vi "CgStop.vi"(3 "error in (no error)":errorcluster, 5 "VISA resource name":refnum<visa-resource-name>) -> (0 "error out":errorcluster, 2 "VISA resource name out":refnum<visa-resource-name>)   [LabVIEW 2009]
doc: "Stops streaming mode of the cyberglove. Also clears any brewing problems with input (at least mostly). Turns light off as well to signal that it is not recording."
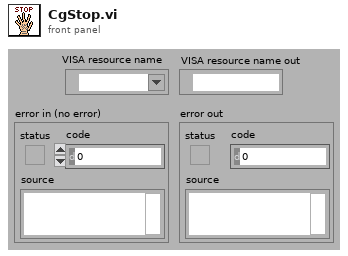
[diagram p1: front panel]
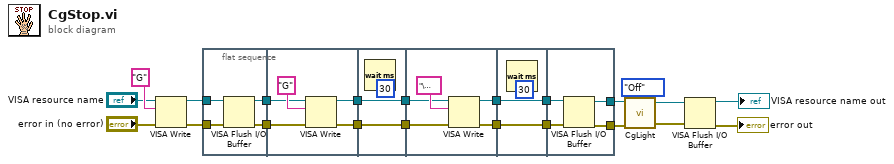
[diagram p0: block diagram]
diagram:
  n1 = VISA Write(VISA resource name="VISA resource name", write buffer="G", error in (no error)="error in (no error)") -> (VISA resource name out=w14:refnum<visa-resource-name>, error out=w13:errorcluster)  [unwired: 1 out]
  n2 = flat-sequence {
    tunnel: w14 -> [w26]
    tunnel: w13 -> [w25]
    tunnel: [w24] -> w12
    tunnel: [w23] -> w11
    tunnel: w12 -> [w30]
    tunnel: w11 -> [w29]
    tunnel: [w28] -> w9
    tunnel: [w27] -> w7
    tunnel: [w33] -> w10
    tunnel: w9 -> [w33]
    tunnel: [w32] -> w8
    tunnel: w7 -> [w32]
    tunnel: w10 -> [w38]
    tunnel: w8 -> [w37]
    tunnel: [w36] -> w5
    tunnel: [w35] -> w3
    tunnel: [w41] -> w6
    tunnel: w5 -> [w41]
    tunnel: [w40] -> w4
    tunnel: w3 -> [w40]
    tunnel: [w46] -> w2
    tunnel: [w45] -> w1
    tunnel: w6 -> [w44]
    tunnel: w4 -> [w43]
    frame #0 {
      n3 = VISA Flush I/O Buffer(VISA resource name=w26, error in (no error)=w25) -> (VISA resource name out=w24:refnum<visa-resource-name>, error out=w23:errorcluster)  [unwired: 1 in]
    }
    frame #1 {
      n4 = VISA Write(VISA resource name=w30, write buffer="G", error in (no error)=w29) -> (VISA resource name out=w28:refnum<visa-resource-name>, error out=w27:errorcluster)  [unwired: 1 out]
    }
    frame #2 {
      n5 = Wait (ms)(milliseconds to wait=u32 30) -> ()  [unwired: 1 out]
    }
    frame #3 {
      n6 = VISA Write(VISA resource name=w38, write buffer="\u0003", error in (no error)=w37) -> (VISA resource name out=w36:refnum<visa-resource-name>, error out=w35:errorcluster)  [unwired: 1 out]
    }
    frame #4 {
      n7 = Wait (ms)(milliseconds to wait=u32 30) -> ()  [unwired: 1 out]
    }
    frame #5 {
      n8 = VISA Flush I/O Buffer(VISA resource name=w44, error in (no error)=w43) -> (VISA resource name out=w46:refnum<visa-resource-name>, error out=w45:errorcluster)  [unwired: 1 in]
    }
  }
  n9 = call "CgLight.vi"("error in (no error)"=w1, "Mode"=enum16{"Off", "On", "Flash"}."Off", "VISA resource name"=w2) -> ("error out"=w17:errorcluster, "VISA resource name out"=w18:refnum<visa-resource-name>)  [unwired: 2 in]
  n10 = VISA Flush I/O Buffer(VISA resource name=w18, error in (no error)=w17) -> (VISA resource name out=→"VISA resource name out":refnum<visa-resource-name>, error out=→"error out":errorcluster)  [unwired: 1 in]
